vi "Coerce Motor Velocities.vi"(11 "Robot Velocities in":T1) -> (3 "Robot Velocities out":T1)   [LabVIEW 2012]
uses:
  Globals.vi
panel:
  in  "IR Panic Range":dbl=0.15
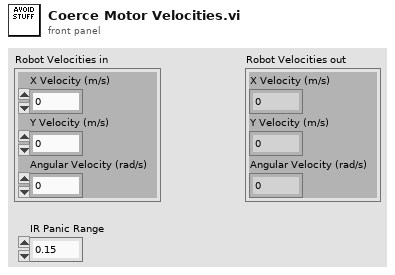
[diagram p1: front panel]
types:
  T1 = cluster{"X Velocity (m/s)":dbl, "Y Velocity (m/s)":dbl, "Angular Velocity (rad/s)":dbl}
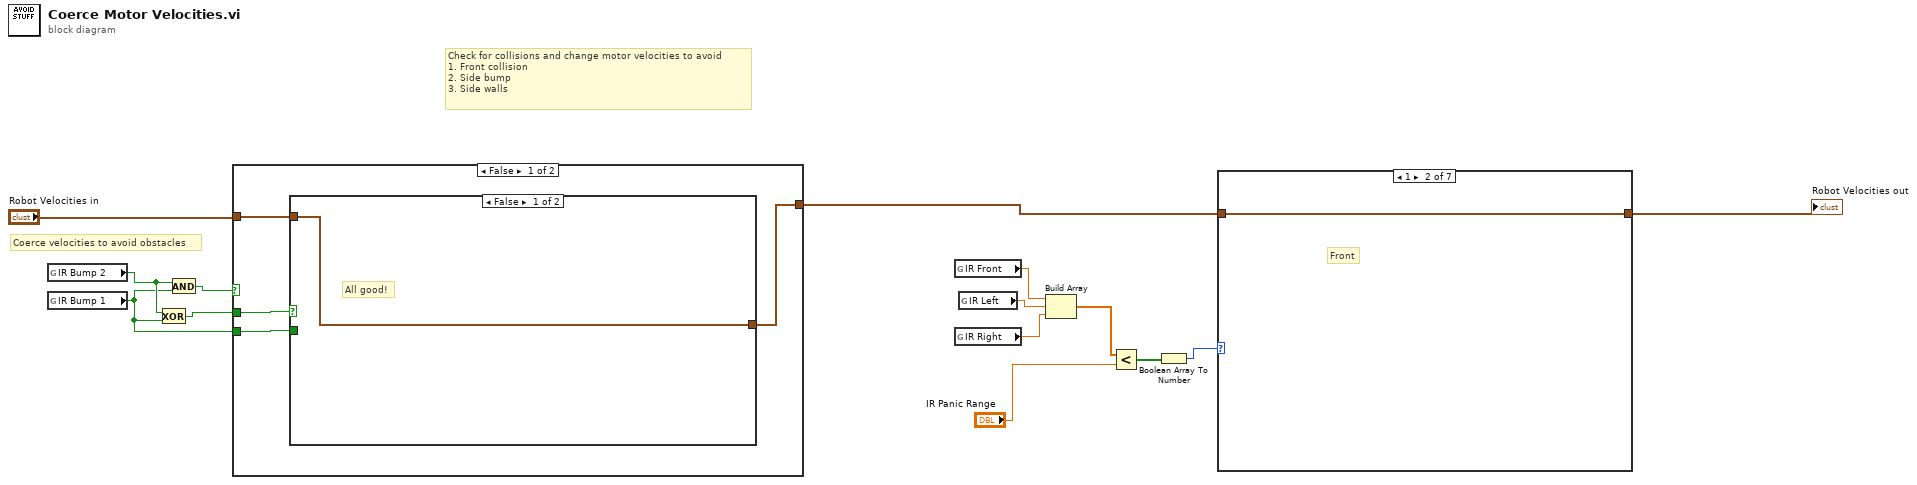
[diagram p0: block diagram]
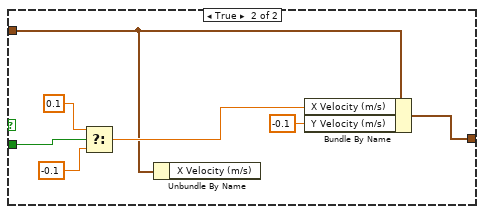
[diagram p8: hidden frame]
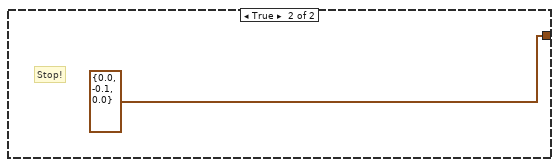
[diagram p9: hidden frame]
diagram:
  # "Check for collisions and change motor velocities to avoid\n1. Front collision\n2. Side bump\n3. Side walls"
  # "Coerce velocities to avoid obstacles"
  n1 = global read "Globals.vi" "IR Bump 2"() -> (w12:bool)
  n2 = global read "Globals.vi" "IR Bump 1"() -> (w11:bool)
  n3 = Exclusive Or(1:w11, 2:w12) -> (0:w13:bool)
  n4 = And(x=w12, y=w11) -> (x .and. y?=w14:bool)
  n5 = case shown="False" w14 {
    tunnel: w13 -> [w18 _]
    tunnel: w11 -> [w17 _]
    tunnel: "Robot Velocities in" -> [w16 _]
    tunnel: [w15 T1 {"X Velocity (m/s)"=0.0, "Y Velocity (m/s)"=-0.1, "Angular Velocity (rad/s)"=0.0} ("Robot Velocities")] -> w9
    frame False {
      n6 = case shown="False" w18 {
        tunnel: w17 -> [_ w26]
        tunnel: w16 -> [w19 w22]
        tunnel: [w19 w21] -> w15
        frame False {
          # "All good!"
        }
        frame True {
          n7 = Select(t=0.1, s=w26, f=-0.1) -> (s? t:f=w25:dbl)
          n8 = Unbundle By Name(w22) -> ()  [unwired: 1 out]
          n9 = Bundle By Name(cluster=w22, "X Velocity (m/s)"=w25, "Y Velocity (m/s)"=-0.1) -> (w21:T1)
        }
      }
    }
    frame True {
      # "Stop!"
    }
  }
  n10 = global read "Globals.vi" "IR Front"() -> (w7:dbl)
  n11 = global read "Globals.vi" "IR Right"() -> (w5:dbl)
  n12 = global read "Globals.vi" "IR Left"() -> (w6:dbl)
  n13 = Build Array(w7, w6, w5) -> (w4:dbl[])
  n14 = Less?(x=w4, y="IR Panic Range") -> (x < y?=w2:bool[])
  n15 = Boolean Array To Number(Boolean array=w2) -> (number=w1:u32)
  n16 = case shown="1" w1 {
    tunnel: [w28 w29 w30 w31 w32 w33 w34] -> w8
    tunnel: w9 -> [w28 w29 w30 w31 w32 w33 w34]
    frame 0, Default {
      # "All good"
    }
    frame 1 {
      # "Front"
    }
    frame 2 {
      # "Left only"
    }
    frame 3 {
      # "Front and left"
    }
    frame 4 {
      # "Right only"
    }
    frame 5 {
      # "Right and front"
    }
    frame 6 {
      # "Left and right"
    }
  }
  "Robot Velocities out" <- w8
